vi "Maintain Field.vi"(8 "error in":errorcluster, 10 "Desired field":dbl[unit], 11 "varian in":refnum<class "Varian Magnet.lvclass">) -> (0 "error out":errorcluster, 1 "Current field":dbl[unit], 2 "At field and stable?":bool, 3 "varian out":refnum<class "Varian Magnet.lvclass">)   [LabVIEW 2009, in "Varian Magnet.lvclass"]
uses:
  Varian Magnet.lvclass
  Varian Magnet.lvclass/Varian Magnet.ctl
  Varian Max Field.vi
  <vilib>/DAQmx/create/channels.llb/DAQmx Create Channel (AO-Voltage-Basic).vi
  Varian/Varian.lvlib
panel:
  out "Waveform Chart":dbl[unit](graph)
  in  "Enum":enum16{"Please Select a Value", "30V", "40V"}(ring)=enum."30V"
  out "Current control voltage":dbl
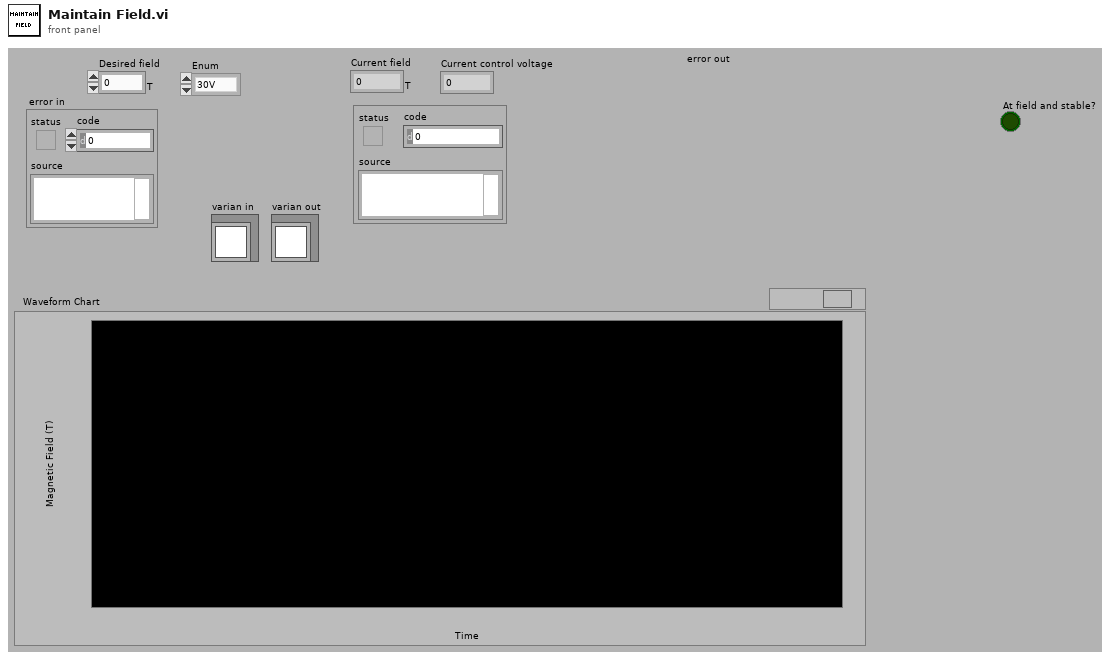
[diagram p1: front panel]
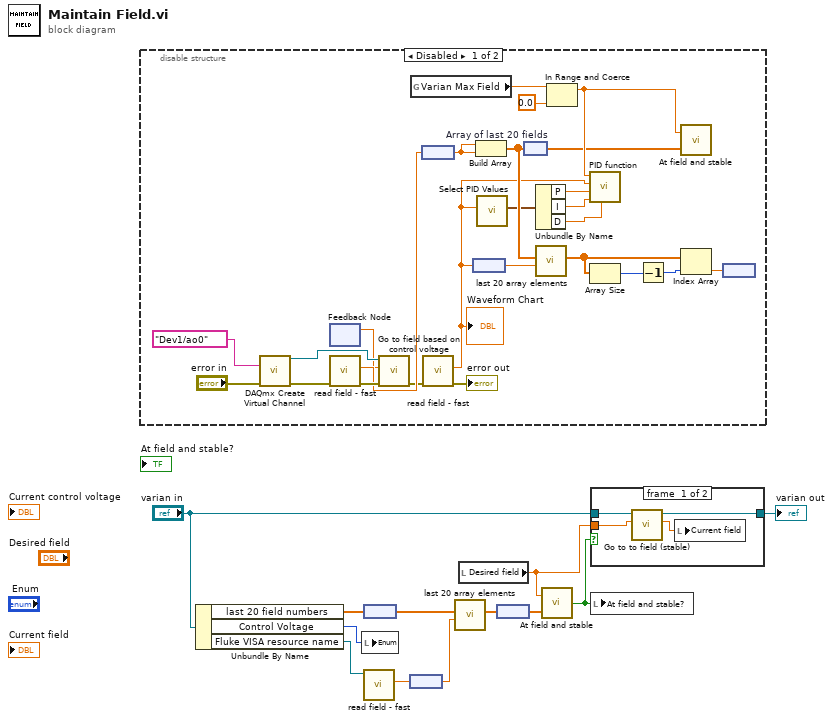
[diagram p0: block diagram]
diagram:
  n1 = disable-structure shown="Disabled" {
    frame #0 {
      n2 = call-poly <vilib>:"DAQmx Create Virtual Channel.vi"("physical channels"=tag "Dev1/ao0", "error in"="error in") -> ("task out"=w36:refnum<k21>, "error out"=w33:errorcluster)  [unwired: 7 in, 5 out]
      n3 = feedback #1() -> (w13:dbl)  [unwired: 1 in]
      n4 = call "read field - fast.vi"("error in (no error)"=w33) -> ("error out"=w38:errorcluster, "Current field (T)"=w37:dbl[unit])  [unwired: 1 in, 8 out]
      n5 = call "Go to field based on control voltage.vi"("error in"=w38, "Control Voltage"=w13, "task in"=w36) -> ("error out"=w22:errorcluster)  [unwired: 8 out]
      n6 = global read "Varian Max Field.vi" "Varian Max Field"() -> (w34:dbl[unit])
      n7 = node(w37) -> (w29:dbl)
      n8 = call "read field - fast.vi"("error in (no error)"=w22) -> ("error out"=→"error out":errorcluster, "Current field (T)"=w16:dbl[unit])  [unwired: 1 in, 8 out]
      "Waveform Chart" <- w16
      n9 = node(w16) -> (w21:dbl)
      n10 = Build Array(w29, w29) -> (w30:dbl[])
      n11 = call "Select PID Values.vi"("current field"=w16) -> ("PID output"=w20:cluster{"I":dbl, "D":dbl, "P":dbl})  [unwired: 9 in, 1 out]
      n12 = node "Array of last 20 fields"(w30) -> (w23:dbl[unit][])
      n13 = Unbundle By Name(w20) -> ("P"=w19:dbl, "I"=w18:dbl, "D"=w17:dbl)
      n14 = call "last 20 array elements.vi"("number to be inserted at end"=w21, "input array"=w30) -> ("output array"=w28:dbl[])  [unwired: 9 out]
      n15 = In Range and Coerce(upper limit=w34, lower limit=dbl[unit] 0.0) -> (coerced(x)=w39:dbl[unit])  [unwired: 1 in, 1 out]
      n16 = call "PID function.vi"("D"=w17, "I"=w18, "P"=w19, "Current Field"=w16, "Field Desired"=w39) -> ("Numeric"=w14:dbl)  [unwired: 6 out]
      n17 = Array Size(array=w28) -> (size(s)=w27:i32)
      n18 = Decrement(x=w27) -> (x-1=w26:i32)
      n19 = call "At field and stable.vi"("last 20 field numbers"=w23, "Desired field"=w39) -> ("At field and stable?"=w15:bool)
      n20 = Index Array(array=w28, index=w26) -> (element=w25:dbl)
      n21 = node(w25) -> ()  [unwired: 1 out]
    }
    frame #1 {
    }
  }
  n22 = Unbundle By Name("varian in") -> ("last 20 field numbers"=w9:dbl[unit][], "Control Voltage"=w2:enum16{"Please Select a Value", "30V", "40V"}, "Fluke VISA resource name"=w1:refnum<visa-resource-name>)
  n23 = local write "Enum"(w2) -> ()
  n24 = node(w9) -> (w8:dbl[])
  n25 = call "read field - fast.vi"("VISA resource name"=w1) -> ("Current field (T)"=w11:dbl[unit])  [unwired: 1 in, 9 out]
  n26 = node(w11) -> (w10:dbl)
  n27 = call "last 20 array elements.vi"("number to be inserted at end"=w10, "input array"=w8) -> ("output array"=w7:dbl[])  [unwired: 9 out]
  n28 = local read "Desired field"() -> (w12:dbl[unit])
  n29 = node(w7) -> (w6:dbl[unit][])
  n30 = call "At field and stable.vi"("last 20 field numbers"=w6, "Desired field"=w12) -> ("At field and stable?"=w3:bool)
  n31 = case shown="False" w3 {
    tunnel: w12 -> [w43 _]
    tunnel: "varian in" -> [w41 w44]
    tunnel: [w40 w44] -> w4
    frame #0 {
      n32 = call "Go to to field (stable).vi"("Desired field"=w43, "varian in"=w41) -> ("Current field"=w42:dbl[unit], "varian out"=w40:refnum<class "Varian Magnet.lvclass">)  [unwired: 6 in, 2 out]
      n33 = local write "Current field"(w42) -> ()
    }
    frame #1 {
    }
  }
  "varian out" <- w4
  n34 = local write "At field and stable?"(w3) -> ()
